vi "FGV stop (old).vi"(8 "error in (no error)":errorcluster, 10 "Stop Input":bool, 11 "States":enum16{"Read", "Write", "Init"}(ring)) -> (0 "error out":errorcluster, 3 "stop Output":bool)   [LabVIEW 2018]
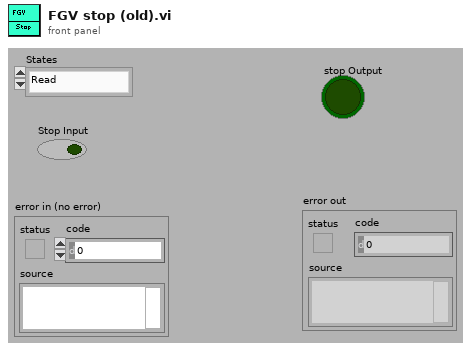
[diagram p1: front panel]
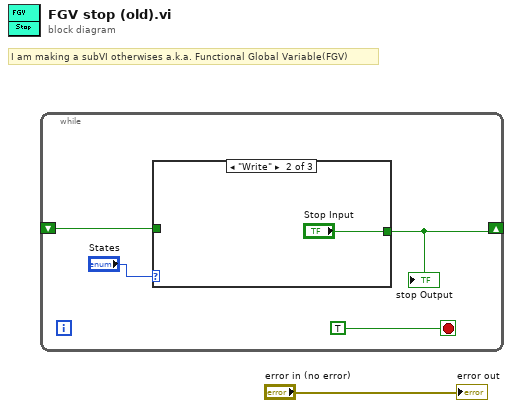
[diagram p0: block diagram]
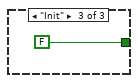
[diagram p3: hidden frame]
diagram:
  # "I am making a subVI otherwises a.k.a. Functional Global Variable(FGV)"
  n1 = while {
    shift-right: [w3] -> _
    shift-left: _ -> [w2]
    stop <- TRUE ("stop") stop-if-true
    n2 = case shown="\"Write\"" "States" {
      tunnel: [w6 "Stop Input" FALSE ("stop")] -> w3
      tunnel: w2 -> [w6 _ _]
      frame "Read", Default {
      }
      frame "Write" {
      }
      frame "Init" {
      }
    }
    "stop Output" <- w3
  }
  "error out" <- "error in (no error)"
